vi "Prepare Self-address.vi"(8 "error in (no error)":errorcluster, 9 "Reply to me":refnum<class "Result Reply Msg.lvclass">, 10 "Reply to":refnum<class "Result Reply Msg.lvclass">, 11 "Process Controller in":refnum<class "Process Controller.lvclass">) -> (0 "error out":errorcluster, 1 "Reply to me":refnum<class "Result Reply Msg.lvclass">, 2 "Active measurements enqueuers":refnum<class "Message Enqueuer.lvclass">[](array[class]), 3 "Process Controller out":refnum<class "Process Controller.lvclass">)   [LabVIEW 2019, in "Process Controller.lvclass"]
uses:
  Process Controller.lvclass
  C:/GitHub/LabActor/Worker/Worker.lvclass
  C:/GitHub/LabActor/Template Module/Template Module.lvclass
  C:/Program Files/National Instruments/LabVIEW 2019/vi.lib/ActorFramework/Actor/Actor.lvclass
  Template Module Messages/Result Reply Msg/Result Reply Msg.lvclass
  C:/GitHub/LabActor/Template Module Messages/Self-Addressed Msg/Self-addressed Msg.lvclass
  <vilib>/ActorFramework/Message Enqueuer/Message Enqueuer.lvclass
  Worker/Worker.lvclass/Worker.ctl
  Template Module/Template Module.lvclass/Template Module.ctl
  <vilib>/ActorFramework/Actor/Actor.lvclass/Actor.ctl
  <vilib>/ActorFramework/Message Enqueuer/Message Enqueuer.lvclass/Message Enqueuer.ctl
  Template Module Messages/Self-Addressed Msg/Self-addressed Msg.lvclass/Self-addressed Msg.ctl
  Process Controller.lvclass/Process Controller.ctl
  Worker/Write Cycle count.vi
  Template Module/Write Reply to.vi
  Template Module Messages/Self-Addressed Msg/Write Return Enqueuer.vi
  <vilib>/ActorFramework/Message Enqueuer/Init from Existing Queue.vi
  <vilib>/ActorFramework/Actor/Actor.lvclass
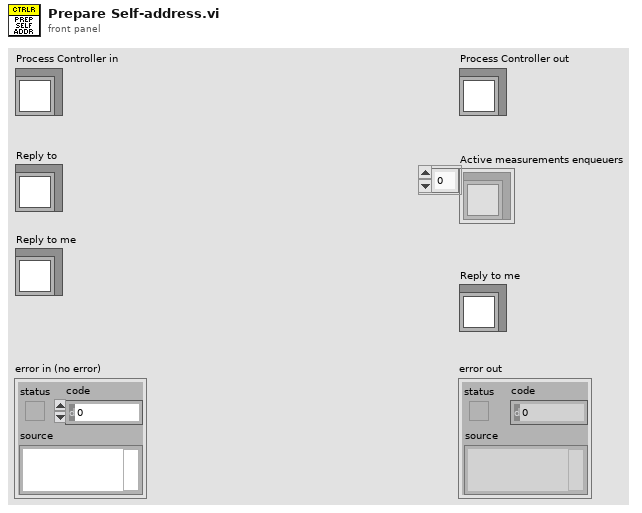
[diagram p1: front panel]
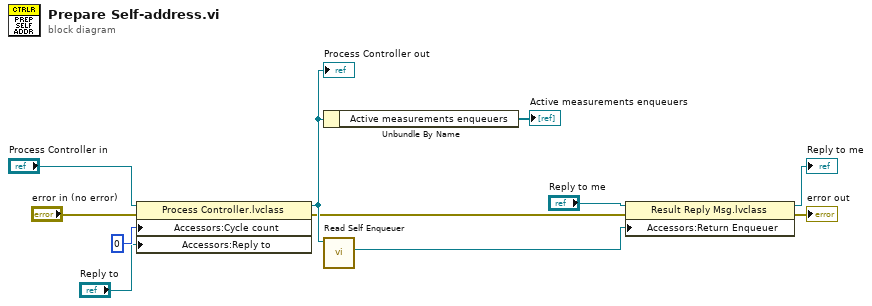
[diagram p0: block diagram]
diagram:
  n1 = property class="Process Controller.lvclass"(reference="Process Controller in", error in="error in (no error)", "Accessors:Cycle count"=0 ("Counter"), "Accessors:Reply to"="Reply to") -> (reference out=w8:refnum<class "Process Controller.lvclass">, error out=w2:errorcluster)
  "Process Controller out" <- w8
  n2 = Unbundle By Name(w8) -> ("Active measurements enqueuers"=→"Active measurements enqueuers":refnum<class "Message Enqueuer.lvclass">[])
  n3 = call <vilib>:"Read Self Enqueuer.vi"("Actor"=w8) -> ("Self Enqueuer"=w6:refnum<class "Message Enqueuer.lvclass">)  [unwired: 10 in]
  n4 = property class="Result Reply Msg.lvclass"(reference="Reply to me", error in=w2, "Accessors:Return Enqueuer"=w6) -> (reference out=→"Reply to me":refnum<class "Result Reply Msg.lvclass">, error out=→"error out":errorcluster)
